vi "From JSON String.vi"() -> ()   [LabVIEW 2017, in "LVJSON.lvlib"]
uses:
  LVJSON.lvlib
  Token Types.ctl
panel:
  out "Value Tokens":cluster{"Token Type":T1, "Token Value":string}[](array[cluster])
  in  "JSON String":string
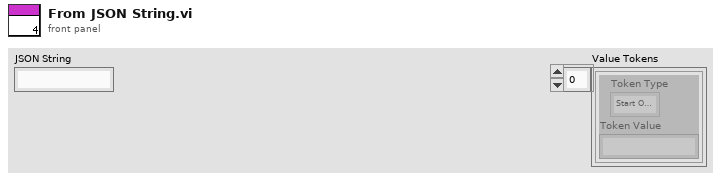
[diagram p1: front panel]
types:
  T1 = typedef "Token Types.ctl" = enum32{"Start Object", "End Object", "Start Array", "End Array", "Colon", "Comma", "Numeric", "true", "false", "null", "String"}
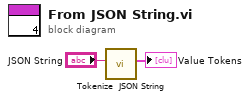
[diagram p0: block diagram]
diagram:
  n1 = call "Tokenize  JSON String.vi"("JSON String"="JSON String") -> ("Value Tokens"=→"Value Tokens":cluster{"Token Type":T1, "Token Value":string}[])  [unwired: 10 in]
